vi "Read Measurement(Math).vi"(0 "VISA resource name":refnum<visa-resource-name>, 5 "Trigger Count (1)":dbl=1.0 format="%#.6g", 7 "Maximum Time (10000ms)":u32=10000, 11 "error in (no error)":errorcluster) -> (3 "Maximum":dbl, 4 "VISA resource name out":refnum<visa-resource-name>, 6 "Count":dbl, 8 "Average":dbl, 10 "Standard Deviation":dbl, 14 "Minimum":dbl, 15 "error out":errorcluster)   [LabVIEW 2013, in "Agilent 3458.lvlib"]
doc: "Takes several measurements and returns statisical analysis of these measurements. Note that the instrument starts taking measurements after setting the trigger count except in cases of external or level triggering in which case it waits for the specified input signal. Set an adequate amount in the Maximum Time control to give the DMM enough time to acquire all measurements. The greater the amount of measurements, then the greater the maximum time will be."
uses:
  Agilent 3458.lvlib
  Low Level/Fetch Measurement(Math).vi
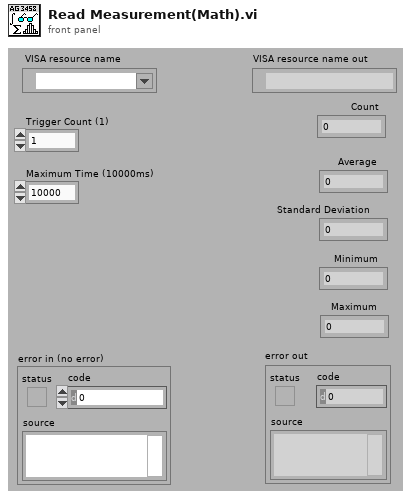
[diagram p1: front panel]
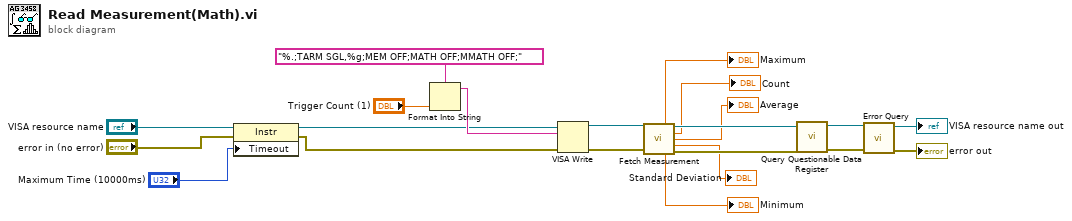
[diagram p0: block diagram]
diagram:
  n1 = property class="Instr"(reference="VISA resource name", error in="error in (no error)", "Timeout"="Maximum Time (10000ms)") -> (reference out=w15:refnum<visa-resource-name>, error out=w14:errorcluster)
  n2 = Format Into String(format string="%.;TARM SGL,%g;MEM OFF;MATH OFF;MMATH OFF;", "Trigger Count (1)") -> (resulting string=w16:string)  [unwired: 2 in, 1 out]
  n3 = VISA Write(VISA resource name=w15, write buffer=w16, error in (no error)=w14) -> (VISA resource name out=w13:refnum<visa-resource-name>, error out=w12:errorcluster)  [unwired: 1 out]
  n4 = call-poly "Fetch Measurement.vi"("VISA resource name"=w13, "error in (no error)"=w12) -> ("Maximum"=→"Maximum":dbl, "VISA resource name out"=w11:refnum<visa-resource-name>, "Count"=→"Count":dbl, "Average"=→"Average":dbl, "Standard Deviation"=→"Standard Deviation":dbl, "Minimum"=→"Minimum":dbl, "error out"=w10:errorcluster)  [unwired: 7 in]
  n5 = call "Query Questionable Data Register.vi"("error in (no error)"=w10, "VISA resource name"=w11) -> ("error out"=w8:errorcluster, "VISA resource name out"=w9:refnum<visa-resource-name>)  [unwired: 7 in, 1 out]
  n6 = call "Error Query.vi"("error in (no error)"=w8, "VISA resource name"=w9) -> ("error out"=→"error out":errorcluster, "VISA resource name out"=→"VISA resource name out":refnum<visa-resource-name>)  [unwired: 6 in, 2 out]
